vi "03. Native MQTT Service Provider.vi"() -> ()   [LabVIEW 2019]
uses:
  Actor/Request -- cluster.ctl
  <vilib>/LabVIEW Open Source Project/MQTT Control Packets/Control Packets/ControlPacket/ControlPacket.lvclass/ControlPacket.ctl
  d83398bf-d288-4447-9c56-1851baa950d7.vi
  3288b219-43a6-48ac-a265-cf9a9541cd0b.vi
  <vilib>/LabVIEW Open Source Project/MQTT Control Packets/Control Packets/PUBLISH/PUBLISH.lvclass
  C:/Program Files (x86)/National Instruments/LabVIEW 2019/vi.lib/LabVIEW Open Source Project/MQTT Control Packets/Control Packets/ControlPacket/ControlPacket.lvclass
  <vilib>/JDP Science/JSONtext/JSON text to Variant.vi
  <vilib>/Utility/error.llb/Error Cluster From Error Code.vi
  <vilib>/JDP Science/JSONtext/LVClass Serializer/JSONtext LVClass Serializer.lvclass
  <vilib>/ErrorRing/Error Ring.xnode
  <vilib>/LabVIEW Open Source Project/MQTT Control Packets/Control Packets/ControlPacket/ControlPacket.lvclass
  <vilib>/JDP Science/JSONtext/JSONtext.lvlib
panel:
  out "<JSON>Response":string
  out "<JSON>":string caption="<JSON>Request"
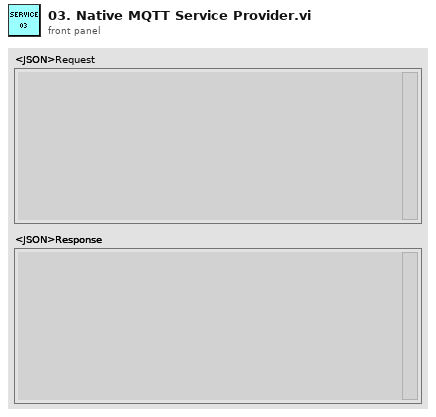
[diagram p1: front panel]
types:
  T1 = typedef "Actor Private Data.ctl" = cluster{"Client":refnum<class "Client.lvclass">, "QualifiedName":string, "EventReg":refnum<event-registration>, "Private Events":T2}
  T2 = typedef "Actor Private Events -- cluster.ctl" = cluster{"Stop":refnum<user-event>, "Subscribe":refnum<user-event>, "Unsubscribe":refnum<user-event>, "publish":refnum<user-event>}
  T3 = typedef "Request -- cluster.ctl" = cluster{"method":string, "<JSON>params":string, "id":string, "reply-topic":string}
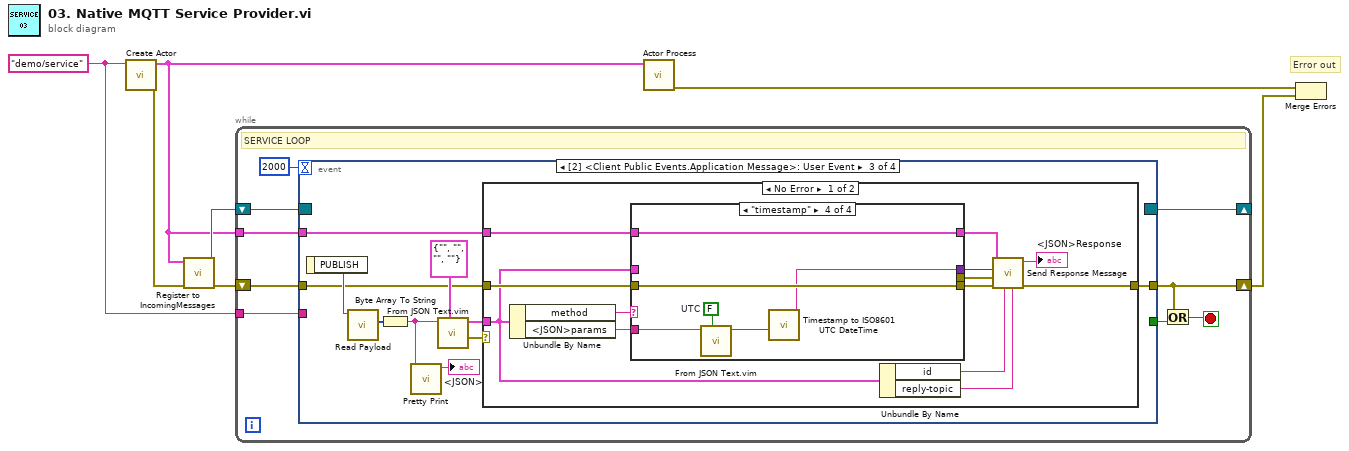
[diagram p0: block diagram]
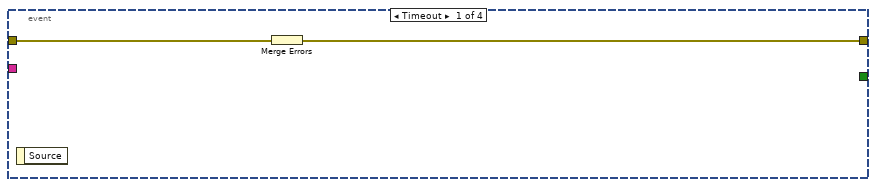
[diagram p2: hidden frame]
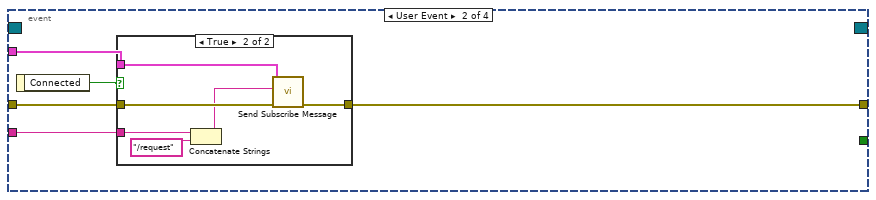
[diagram p3: hidden frame]
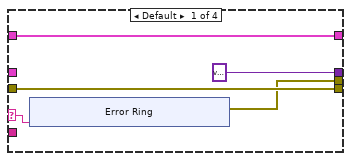
[diagram p5: hidden frame]
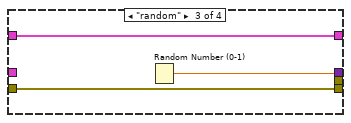
[diagram p7: hidden frame]
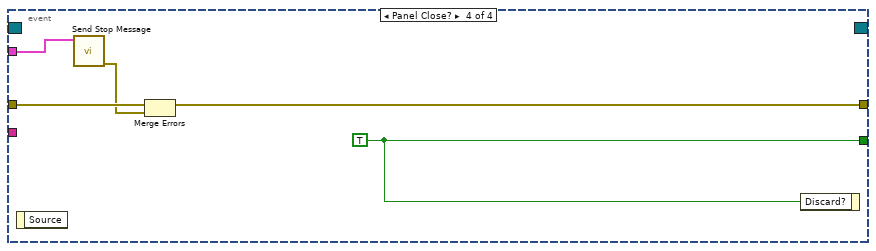
[diagram p9: hidden frame]
diagram:
  w2 = "demo/service" ("QualifiedName")
  # "Error out"
  n1 = call "Create Actor.vi"("QualifiedName"=w2) -> ("error out"=w6:errorcluster, "Actor Class"=w4:T1)  [unwired: 9 in]
  n2 = call "Register to IncomingMessages.vi"("error in"=w6, "Actor Class"=w4) -> ("error out"=w3:errorcluster, "Incoming Messages"=w5:refnum<event-registration>)  [unwired: 8 in]
  n3 = while {
    tunnel: w4 -> [w14]
    shift-right: [w11] -> _
    shift-left: w5 -> [w12]
    shift-right: [w9] -> w1
    shift-left: w3 -> [w10]
    tunnel: w2 -> [w8]
    stop <- w15 stop-if-true
    # "SERVICE LOOP"
    n4 = event shown="[2] <Client Public Events.Application Message>: User Event" {
      selector: w12 -> [_ _ _ _]
      dyn-events: [_ _ _ _] -> w11
      timeout: 2000 -> [_ _ _ _]
      tunnel: [_ _ _ w83] -> w16
      tunnel: w14 -> [_ w21 w35 w82]
      tunnel: [w17 w22 w33 w79] -> w9
      tunnel: w10 -> [w18 w23 w34 w81]
      tunnel: w8 -> [_ w19 _ _]
      event Timeout {
        n5 = event-data() -> ()  [unwired: 1 in, 1 out]
        n6 = Merge Errors(w18) -> (w17:errorcluster)
      }
      event User Event {
        n7 = event-data() -> ("Connected"=w20:bool)  [unwired: 1 in]
        n8 = case shown="True" w20 {
          tunnel: w23 -> [w24 w30]
          tunnel: [w24 w29] -> w22
          tunnel: w21 -> [_ w28]
          tunnel: w19 -> [_ w27]
          frame False {
          }
          frame True {
            n9 = Concatenate Strings(w27, "/request" ("QualifiedName")) -> (w25:string)
            n10 = call "Send Subscribe Message.vi"("error in"=w30, "Topic"=w25, "Actor Class"=w28) -> ("error out"=w29:errorcluster)  [unwired: 8 in]
          }
        }
      }
      event User Event {
        n11 = event-data() -> ("PUBLISH"=w40:refnum<class "PUBLISH.lvclass">)  [unwired: 1 in]
        n12 = call <vilib>:"Read Payload.vi"("ControlPacket in"=w40) -> ("Payload"=w39:u8[])  [unwired: 9 in, 1 out]
        n13 = Byte Array To String(unsigned byte array=w39) -> (string=w32:string)
        n14 = call <vilib>:"Pretty Print.vi"("JSON"=w32) -> ("<JSON>"=→"<JSON>":string)  [unwired: 8 in, 2 out]
        n15 = call "From JSON Text.vim"("Data Type and Default Value"=T3 {"method"="", "<JSON>params"="", "id"="", "reply-topic"=""} ("request"), "JSON"=w32) -> ("error out"=w37:errorcluster, "Data out"=w36:T3)  [unwired: 8 in]
        n16 = case shown="No Error" w37 {
          tunnel: w36 -> [w42 _]
          tunnel: w35 -> [w51 _]
          tunnel: w34 -> [w50 w78]
          tunnel: [w48 w78] -> w33
          frame No Error {
            n17 = Unbundle By Name(w42) -> ("method"=w53:string, "<JSON>params"=w52:string)
            n18 = case shown="\"timestamp\"" w53 {
              selector: w53 -> [w54 _ _ _]
              tunnel: w52 -> [_ _ _ w75]
              tunnel: w51 -> [w57 w67 w70 w76]
              tunnel: w50 -> [w58 w68 w71 w77]
              tunnel: [w58 w68 w71 w77] -> w47
              tunnel: [w57 w67 w70 w76] -> w49
              tunnel: [w56 _ _ _] -> w44
              tunnel: [variant ("result") w66 w69 w72] -> w43
              tunnel: w42 -> [_ w66 _ _]
              frame Default {
                n19 = xnode "Error Ring"("parameter 0"=w54) -> ("error out"=w56:errorcluster)
              }
              frame "echo" {
              }
              frame "random" {
                n20 = Random Number (0-1)() -> (number: 0 to 1=w69:dbl)
              }
              frame "timestamp" {
                w74 = FALSE  # UTC
                n21 = call "From JSON Text.vim"("Data Type and Default Value"=w74, "JSON"=w75) -> ("Data out"=w73:bool)  [unwired: 8 in, 1 out]
                n22 = call <vilib>:"Timestamp to ISO8601 UTC DateTime.vi"("UTC? (F)"=w73) -> ("ISO8601 UTC DateTime"=w72:string)  [unwired: 10 in]
              }
            }
            n23 = Unbundle By Name(w42) -> ("id"=w46:string, "reply-topic"=w45:string)
            n24 = call "Send Response Message.vi"("topic"=w45, "id"=w46, "error in"=w47, "request error"=w44, "result"=w43, "Actor Class"=w49) -> ("error out"=w48:errorcluster, "<JSON>Response"=→"<JSON>Response":string)  [unwired: 4 in]
          }
          frame Error {
            # "Invalid request payload"
          }
        }
      }
      event Panel Close? {
        w83 = TRUE ("Discard?")
        n25 = event-data() -> ()  [unwired: 1 in, 1 out]
        n26 = call "Send Stop Message.vi"("Actor Class"=w82) -> ("error out"=w80:errorcluster)  [unwired: 10 in]
        n27 = Merge Errors(w81, w80) -> (w79:errorcluster)
        n28 = event-data("Discard?"=w83) -> ()  [unwired: 1 in, 1 out]
      }
    }
    n29 = Or(x=w9, y=w16) -> (x .or. y?=w15:bool)
  }
  n30 = call "Actor Process.vi"("Actor Class"=w4) -> ("error out"=w7:errorcluster)  [unwired: 10 in]
  n31 = Merge Errors(w7, w1) -> ()  [unwired: 1 out]
